vi "ce_liang_kuan_du-5.12.vi"(2 "error in":errorcluster) -> (0 "error out":errorcluster, 1 "data":dbl format="%0.2f")   [LabVIEW 2015]
uses:
  <vilib>/DAQmx/read.llb/DAQmx Read (Counter DBL 1Chan 1Samp).vi
  <vilib>/DAQmx/create/channels.llb/DAQmx Create Channel (CI-Pulse Width).vi
  <vilib>/DAQmx/miscellaneous.llb/DAQmx Fill In Error Info.vi
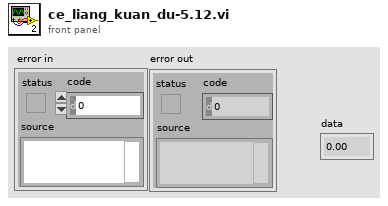
[diagram p1: front panel]
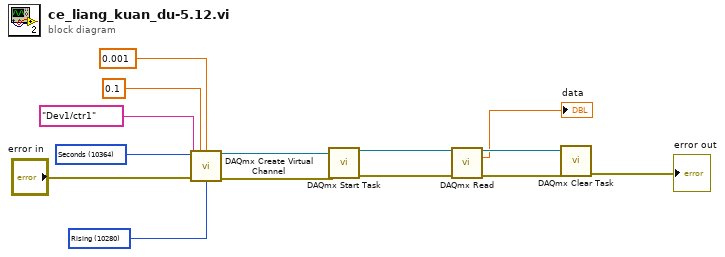
[diagram p0: block diagram]
diagram:
  w10 = 10364 items=["Seconds"=10364, "Ticks"=10304, "From Custom Scale"=10065] ("units")
  w11 = 10280 items=["Rising"=10280, "Falling"=10171] ("starting edge")
  n1 = call-poly <vilib>:"DAQmx Create Virtual Channel.vi"("maximum value"=0.1, "minimum value"=0.001, "counter"=tag "Dev1/ctr1", "units"=w10, "error in"="error in", "starting edge"=w11) -> ("task out"=w8:refnum<k21>, "error out"=w7:errorcluster)  [unwired: 8 in]
  n2 = call <vilib>:"DAQmx Start Task.vi"("task/channels in"=w8, "error in"=w7) -> ("task out"=w6:refnum<k21>, "error out"=w5:errorcluster)  [unwired: 12 in]
  n3 = call-poly <vilib>:"DAQmx Read.vi"("task/channels in"=w6, "error in"=w5) -> ("task out"=w4:refnum<k21>, "data"=→"data":dbl, "error out"=w3:errorcluster)  [unwired: 11 in]
  n4 = call <vilib>:"DAQmx Clear Task.vi"("task in"=w4, "error in"=w3) -> ("error out"=→"error out":errorcluster)  [unwired: 13 in]
